vi "MAC-Tester.vi"() -> ()   [LabVIEW 2017]
uses:
  <vilib>/rvi/interface/nirviMethod/nirviMethod.xnode
  <vilib>/rvi/errors/niLvFpgaMergeErrorWithErrorCode.vi
  <vilib>/rvi/interface/nirviCloseFPGA/nirviCloseFPGA.xnode
  MAC.Events.ctl
  <vilib>/rvi/interface/nirviOpenFPGA/nirviOpenFPGA.xnode
  <vilib>/FPGAPlugInAG/Dynamic/niLvFpga_ReadFifo_Dynamic.vi
  <vilib>/FPGAPlugInAG/Dynamic/niLvFpga_WriteFifo_Dynamic.vi
  FPGA Bitfiles/Fpga-Mac-Top.lvbitx
  Globals.vi
  <vilib>/FPGAPlugInAG/Dynamic/niLvFpga_Close_Dynamic.vi
  <vilib>/FPGAPlugInAG/PXIe-6592R/niLvFpga_Open_PXIe-6592R.vi
  <vilib>/rvi/interface/common/dynamic/niFpgaDynamicAddResources.vi
panel:
  out "IPv4 Header":T1={"Version"=4, "Header Length"=20, "Total Length"=54, "More Fragments"=FALSE, "Don't Fragment"=FALSE, "Fragment Offset"=0, "TTL"=64, "Header Checksum"=58141, "Identification"=16593, "Protocol"=17} {"Header Checksum" format="%04x"}
  in  "IP Address":u8[](array[numeric])=[10, 0, 1, 101]
  in  "MAC":u8[](array[numeric])=[0, 1, 2, 3, 4, 5] format="%.0x"
  in  "Ethernet II Params":T2={"Destination MAC"=[0, 2, 201, 85, 8, 68], "Source MAC"=[0, 1, 2, 3, 4, 5], "EtherType"=2048} {"Destination MAC" format="%.0x"; "Source MAC" format="%.02x"; "EtherType" format="%.0x"}
  in  "IPv4 Params":T3={"Destination IP"=[10, 0, 1, 100], "Source IP"=[10, 0, 1, 101], "Protocol"=17}
  in  "UDP Params":T4={"Source Port"=35312, "Destination Port"=35312, "Payload"="ABCD"}
  out "Status":string
  out "error out":errorcluster
  in  "Exit":bool
  in  "Transmit Packet":bool
  in  "Read Packet":bool
  out "RX Data":u8[](array[numeric])=[0, 1, 2, 3, 4, 5, 0, 2, 201, 85, 8, 68, 8, 6, 0, 1, 8, 0, 6, 4, 0, 1, 0, 2, 201, 85, 8, 68, 10, 0, 1, 100, 0, 0, 0, 0, 0, 0, 10, 0, 1, 101, 0, 0, 0, 0, 0, 0, 0, 0, 0, 0, 0, 0, 0, 0, 0, 0, 0, 0, 28, 161, 25, 173] format="%.0x"
  in  "error in":errorcluster
  # "Send Parameters"
  # "Received Data"
  # "NIC Parameters"
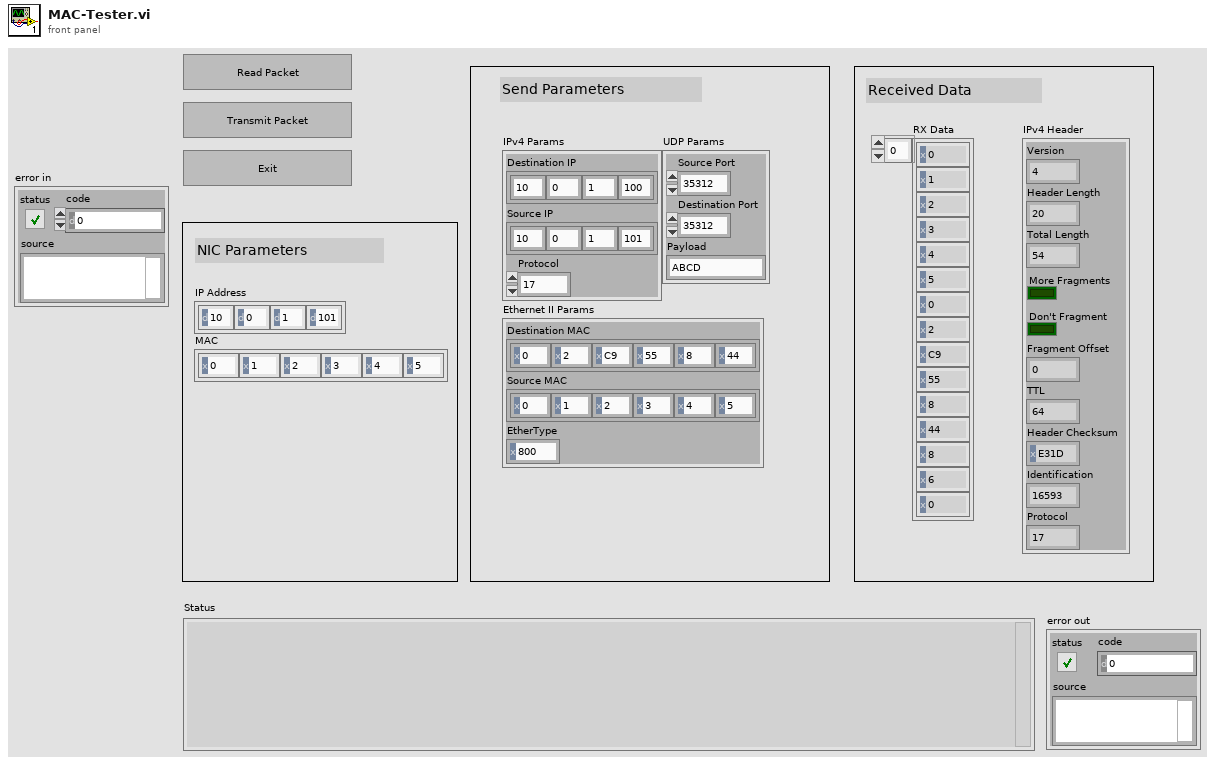
[diagram p1: front panel]
types:
  T1 = cluster{"Version":u8, "Header Length":u8, "Total Length":u16, "More Fragments":bool, "Don't Fragment":bool, "Fragment Offset":u16, "TTL":u8, "Header Checksum":u16, "Identification":u16, "Protocol":u8}
  T2 = cluster{"Destination MAC":u8[], "Source MAC":u8[], "EtherType":u16}
  T3 = cluster{"Destination IP":u8[], "Source IP":u8[], "Protocol":u8}
  T4 = cluster{"Source Port":u16, "Destination Port":u16, "Payload":string}
  T5 = typedef "MAC.Events.ctl" = enum16{"Open FPGA", "Close FPGA", "Poll RX", "Transmit Packet"}
  T6 = cluster{"Version":u8, "Header Length":u8, "Total Length":u16, "More Fragments":bool, "Don't Fragment":bool, "Fragment Offset":u16, "TTL":u8, "Header Checksum":u16, "Identification":u16, "Protocol":u8, "Source IP":u8[], "Destination IP":u8[]}
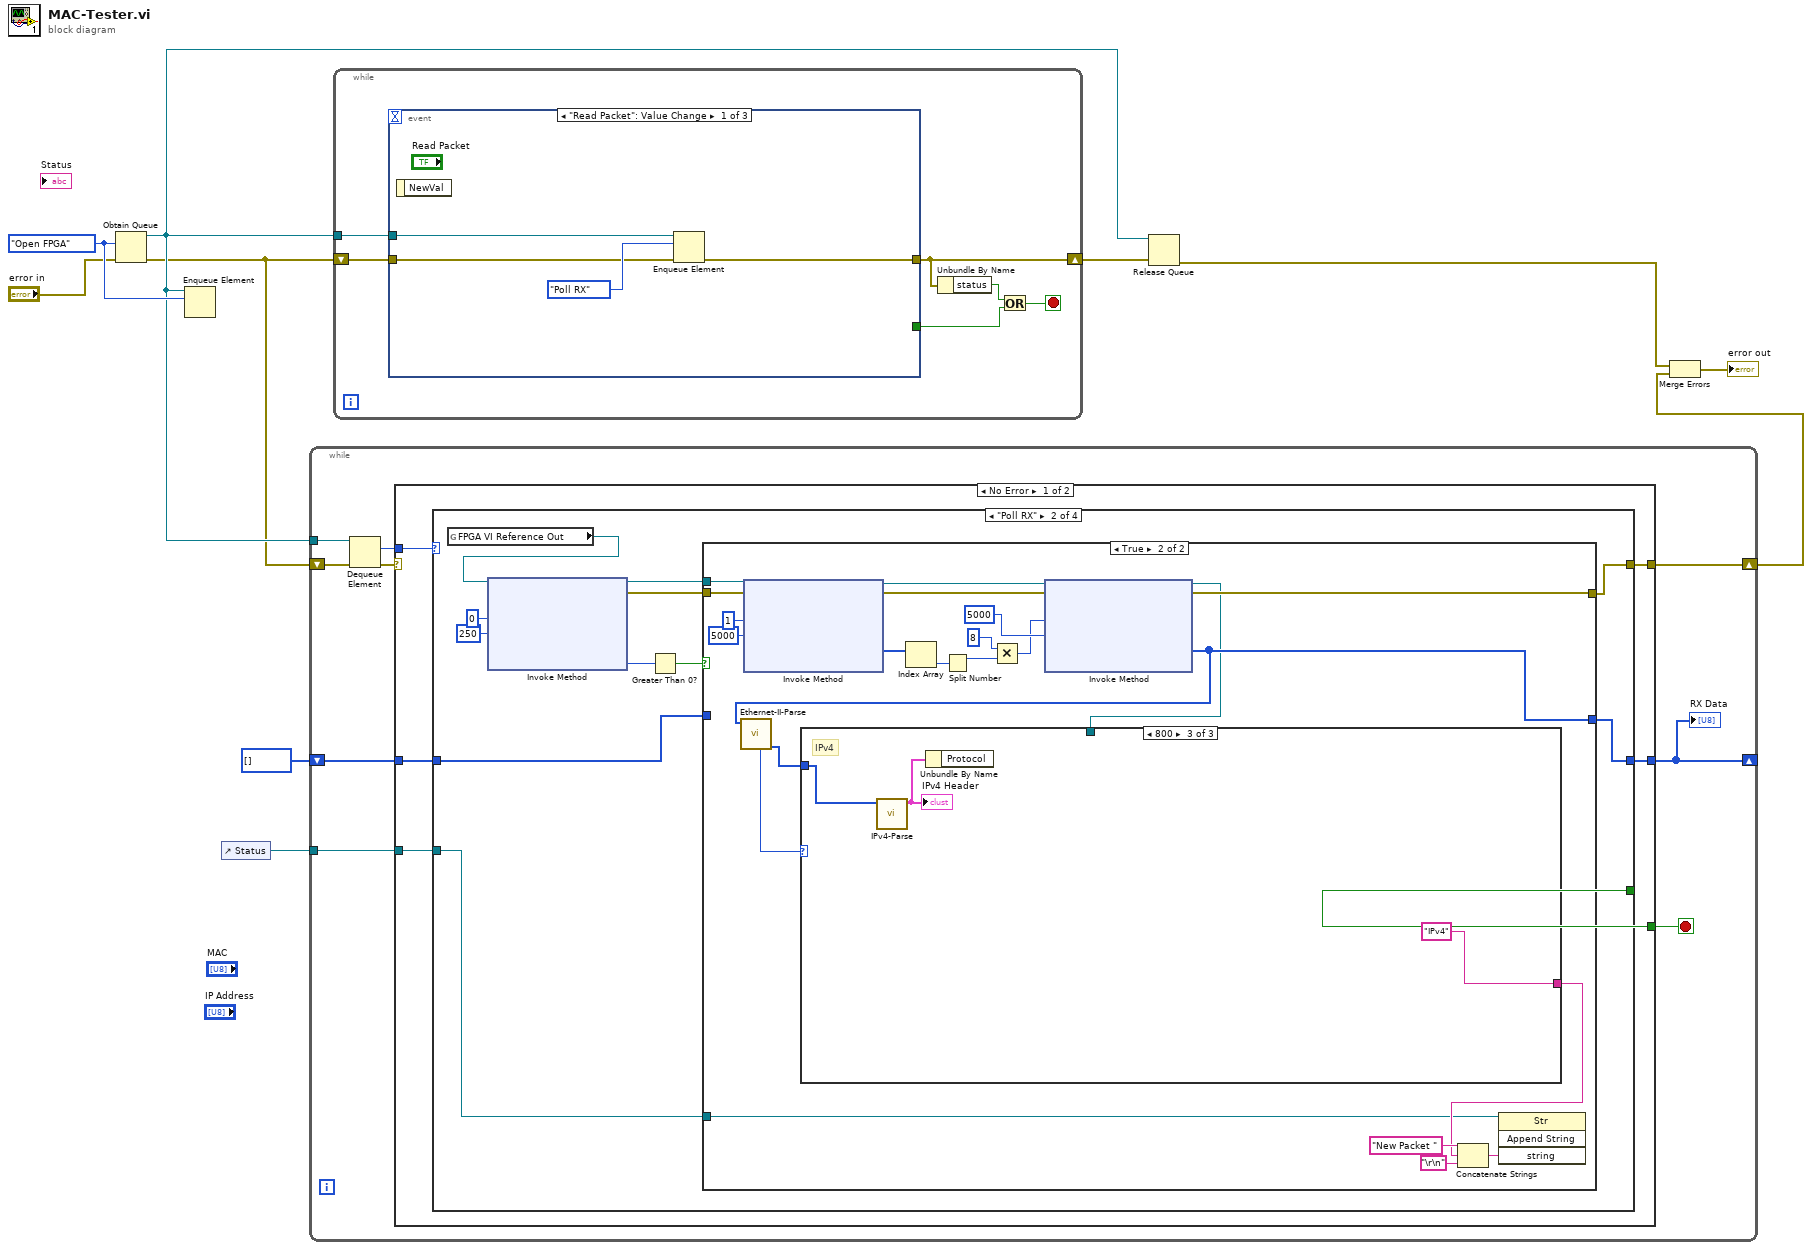
[diagram p0: block diagram]
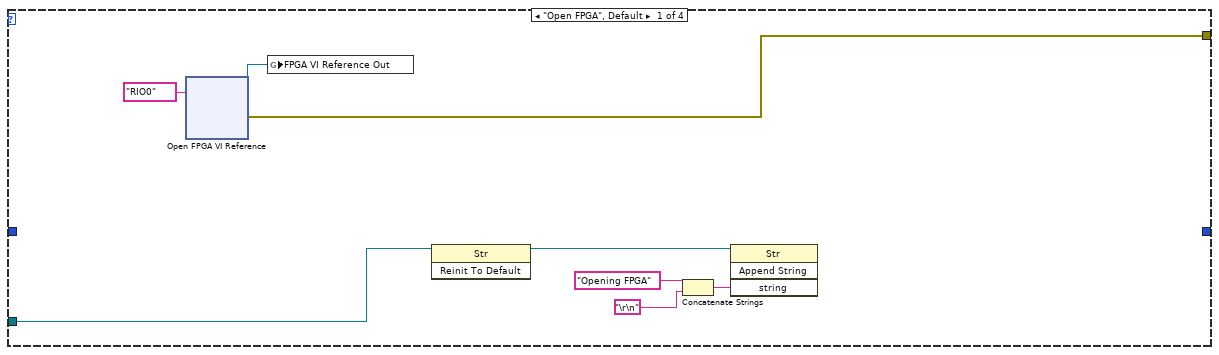
[diagram p2: hidden frame]
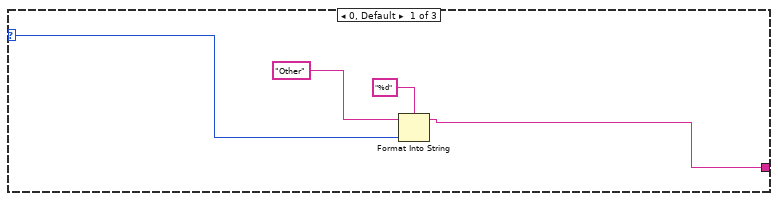
[diagram p4: hidden frame]
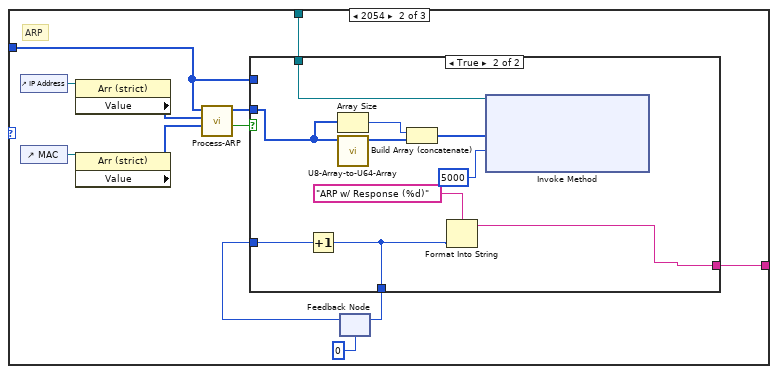
[diagram p5: hidden frame]
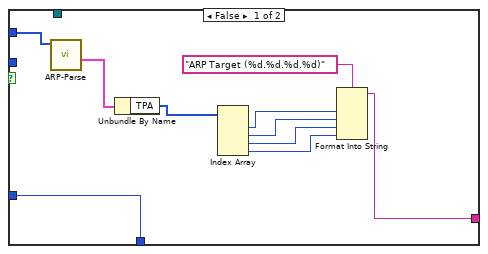
[diagram p6: hidden frame]
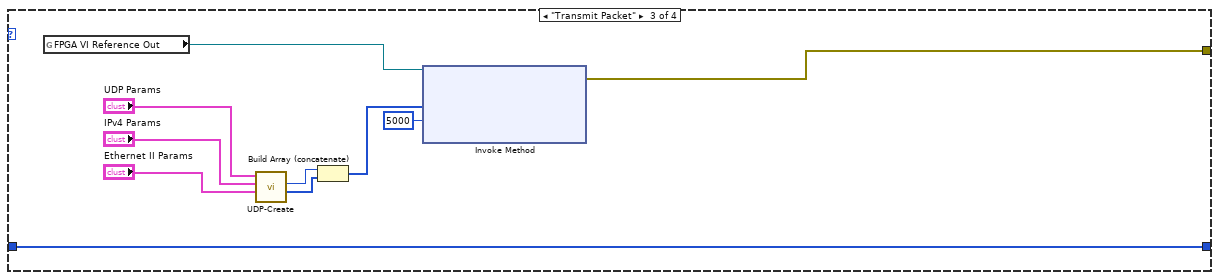
[diagram p7: hidden frame]
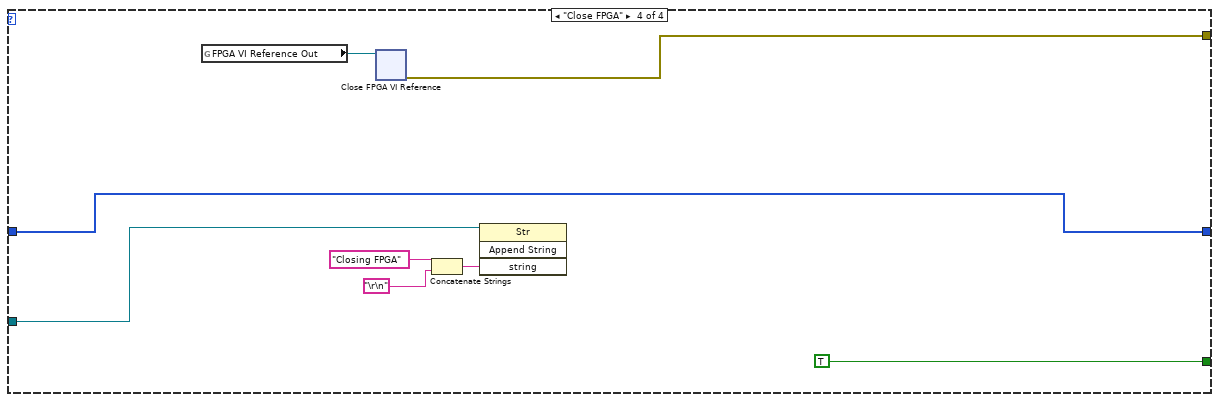
[diagram p8: hidden frame]
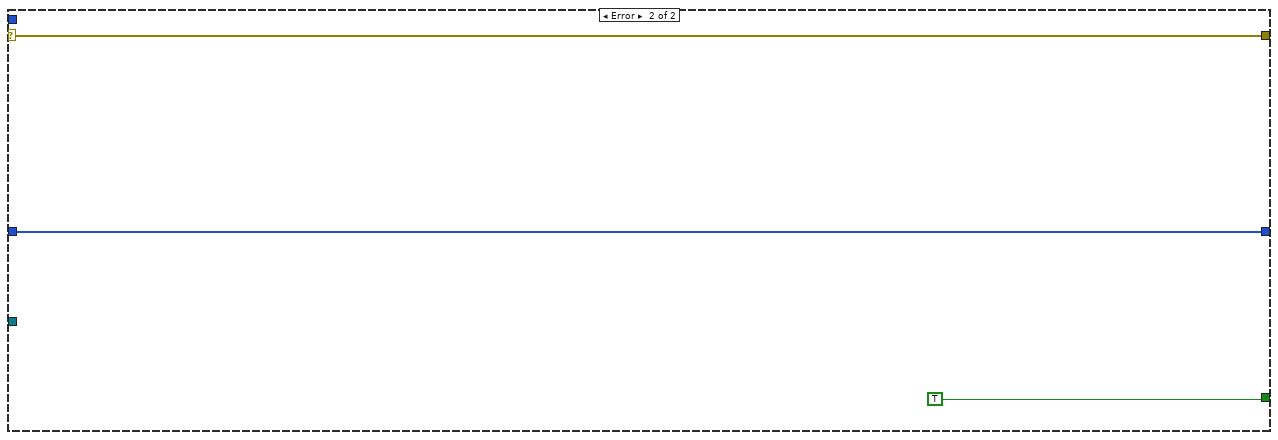
[diagram p9: hidden frame]
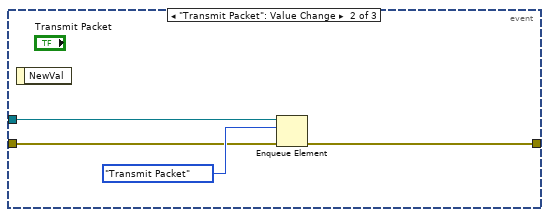
[diagram p10: hidden frame]
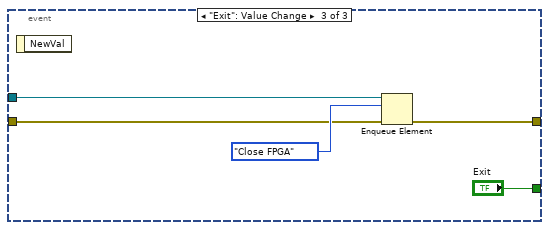
[diagram p11: hidden frame]
diagram:
  w10 = MAC.Events."Open FPGA"
  n1 = Obtain Queue(element data type=w10, error in (no error)="error in") -> (queue out=w8:refnum<queue>, error out=w6:errorcluster)  [unwired: 3 in, 1 out]
  n2 = Enqueue Element(queue=w8, element=w10) -> ()  [unwired: 2 in, 3 out]
  n3 = control-ref of="Status"() -> (w4:refnum<vi>)
  n4 = while {
    tunnel: w8 -> [w19]
    shift-right: [w13] -> w3
    shift-left: w6 -> [w15]
    shift-right: [w12] -> _
    shift-left: u8[] [] -> [w14]
    tunnel: w4 -> [w11]
    stop <- w16 stop-if-true
    n5 = Dequeue Element(queue=w19, error in (no error)=w15) -> (element=w17:T5, error out=w18:errorcluster)  [unwired: 1 in, 2 out]
    n6 = case shown="No Error" w18 {
      selector: w18 -> [_ w126]
      tunnel: w17 -> [w25 _]
      tunnel: [w24 TRUE] -> w16
      tunnel: [w23 w126] -> w13
      tunnel: w14 -> [w22 w127]
      tunnel: [w21 w127] -> w12
      tunnel: w11 -> [w20 _]
      frame No Error {
        n7 = case shown="\"Poll RX\"" w25 {
          tunnel: [_ _ _ TRUE] -> w24
          tunnel: [w33 w36 w109 w124] -> w23
          tunnel: w22 -> [_ w38 w117 w119]
          tunnel: [_ w37 w117 w119] -> w21
          tunnel: w20 -> [w29 w35 _ w120]
          frame "Open FPGA", Default {
            n8 = xnode "Open FPGA VI Reference"("resource name"=tag "RIO0") -> ("FPGA VI Reference Out"=w26:refnum<k20>, "error out"=w33:errorcluster)  [unwired: 1 in]
            n9 = global write "Globals.vi" "FPGA VI Reference Out"(w26) -> ()
            n10 = invoke class="Str" method="Reinit To Default"(reference=w29) -> (reference out=w28:refnum<vi>)  [unwired: 2 in, 2 out]
            n11 = Concatenate Strings("Opening FPGA" ("string"), "\r\n") -> (w32:string)
            n12 = invoke class="Str" method="Append String"(reference=w28, "string"=w32) -> ()  [unwired: 2 in, 4 out]
          }
          frame "Poll RX" {
            n13 = global read "Globals.vi" "FPGA VI Reference Out"() -> (w34:refnum<k20>)
            n14 = xnode "Invoke Method"("FPGA VI Reference In"=w34, "Number of Elements"=u32 0, "Timeout (ms)"=250) -> ("FPGA VI Reference Out"=w40:refnum<k20>, "error out"=w39:errorcluster, "Elements Remaining"=w42:u32)  [unwired: 1 in, 1 out]
            n15 = Greater Than 0?(x=w42) -> (x > 0?=w41:bool)
            n16 = case shown="True" w41 {
              tunnel: w40 -> [_ w66]
              tunnel: w39 -> [w45 w65]
              tunnel: w38 -> [w46 _]
              tunnel: [w46 w50] -> w37
              tunnel: [w45 w59] -> w36
              tunnel: w35 -> [_ w48]
              frame False {
              }
              frame True {
                n17 = xnode "Invoke Method"("FPGA VI Reference In"=w66, "error in"=w65, "Number of Elements"=u32 1, "Timeout (ms)"=5000) -> ("FPGA VI Reference Out"=w62:refnum<k20>, "error out"=w63:errorcluster, "Data"=w64:u32[])  [unwired: 1 out]
                n18 = Index Array(array=w64) -> (element=w61:u32)  [unwired: 1 in]
                n19 = Split Number(x=w61) -> (hi(x)=w55:u16)  [unwired: 1 out]
                n20 = Multiply(x=u16 8 ("y"), y=w55) -> (x*y=w58:u16)
                n21 = xnode "Invoke Method"("FPGA VI Reference In"=w62, "error in"=w63, "Number of Elements"=w58, "Timeout (ms)"=5000) -> ("FPGA VI Reference Out"=w49:refnum<k20>, "error out"=w59:errorcluster, "Data"=w50:u8[])  [unwired: 1 out]
                n22 = call "Ethernet-II-Parse.vi"("Input Frame"=w50) -> ("Payload"=w47:u8[], "EtherType"=w53:u16)  [unwired: 6 in, 3 out]
                n23 = case shown="800" w53 {
                  selector: w53 -> [w72 _ _]
                  tunnel: [w69 w80 "IPv4" ("string")] -> w51
                  tunnel: w47 -> [_ w73 w106]
                  tunnel: w49 -> [_ w77 _]
                  frame 0, Default {
                    n24 = Format Into String(format string="%d", initial string="Other" ("string"), w72) -> (resulting string=w69:string)  [unwired: 1 in, 1 out]
                  }
                  frame 2054 {
                    # "ARP"
                    n25 = control-ref of="IP Address"() -> (w82:refnum<vi>)
                    n26 = control-ref of="MAC"() -> (w84:refnum<vi>)
                    n27 = property class="Arr (strict)"(reference=w82) -> ("Value"=w81:u8[])  [unwired: 1 in, 2 out]
                    n28 = property class="Arr (strict)"(reference=w84) -> ("Value"=w83:u8[])  [unwired: 1 in, 2 out]
                    n29 = call "Process-ARP.vi"(9:w83, "Source Machine\nSettings"=w81, "Frame (in)"=w73) -> ("Response\nNeeded?"=w79:bool, "ARP Response"=w78:u8[])  [unwired: 7 in]
                    n30 = feedback #1(0) -> (w74:i32)
                    n31 = case shown="True" w79 {
                      tunnel: [w91 w95] -> w80
                      tunnel: w78 -> [_ w102]
                      tunnel: w77 -> [_ w103]
                      tunnel: [w94 w97] -> w75
                      tunnel: w74 -> [w94 w98]
                      tunnel: w73 -> [w93 _]
                      frame False {
                        n32 = call "ARP-Parse.vi"("Frame (in)"=w93) -> ("Target"=w90:cluster{"THA":u8[], "TPA":u8[]})  [unwired: 8 in, 2 out]
                        n33 = Unbundle By Name(w90) -> ("TPA"=w89:u8[])
                        n34 = Index Array(array=w89) -> (element #1=w88:u8, element #2=w85:u8, element #3=w86:u8, element #4=w87:u8)  [unwired: 4 in]
                        n35 = Format Into String(format string="ARP Target (%d.%d.%d.%d)", w88, w85, w86, w87) -> (resulting string=w91:string)  [unwired: 2 in, 1 out]
                      }
                      frame True {
                        n36 = Increment(x=w98) -> (x+1=w97:i32)
                        n37 = Array Size(array=w102) -> (size(s)=w100:i32)
                        n38 = call "U8-Array-to-U64-Array.vi"("Frame U8[] in"=w102) -> ("Frame U64[] out"=w101:u64[])  [unwired: 10 in]
                        n39 = Build Array (concatenate)(w100, w101) -> (w99:u64[])
                        n40 = Format Into String(format string="ARP w/ Response (%d)", w97) -> (resulting string=w95:string)  [unwired: 2 in, 1 out]
                        n41 = xnode "Invoke Method"("FPGA VI Reference In"=w103, "Data"=w99, "Timeout (ms)"=5000) -> ()  [unwired: 1 in, 3 out]
                      }
                    }
                    n42 = feedback-in #1(w75) -> ()
                  }
                  frame 2048 {
                    # "IPv4"
                    n43 = call "IPv4-Parse.vi"("IPv4 Packet (in)"=w106) -> ("Header"=w105:T6)  [unwired: 8 in, 2 out]
                    "IPv4 Header" <- w105
                    n44 = Unbundle By Name(w105) -> ()  [unwired: 1 out]
                  }
                }
                n45 = Concatenate Strings("New Packet " ("string"), w51, "\r\n") -> (w57:string)
                n46 = invoke class="Str" method="Append String"(reference=w48, "string"=w57) -> ()  [unwired: 2 in, 4 out]
              }
            }
          }
          frame "Transmit Packet" {
            n47 = global read "Globals.vi" "FPGA VI Reference Out"() -> (w108:refnum<k20>)
            n48 = call "UDP-Create.vi"("Ethernet II Params"="Ethernet II Params", "IPv4 Params"="IPv4 Params", "UDP Params"="UDP Params") -> ("Ethernet Frame\nU64"=w112:u64[], "Ethernet Frame\nsize"=w113:i32)  [unwired: 6 in, 1 out]
            n49 = Build Array (concatenate)(w113, w112) -> (w111:u64[])
            n50 = xnode "Invoke Method"("FPGA VI Reference In"=w108, "Data"=w111, "Timeout (ms)"=5000) -> ("error out"=w109:errorcluster)  [unwired: 1 in, 2 out]
          }
          frame "Close FPGA" {
            n51 = global read "Globals.vi" "FPGA VI Reference Out"() -> (w118:refnum<k20>)
            n52 = xnode "Close FPGA VI Reference"("FPGA VI Reference In"=w118) -> ("error out"=w124:errorcluster)  [unwired: 1 in]
            n53 = Concatenate Strings("Closing FPGA" ("string"), "\r\n") -> (w123:string)
            n54 = invoke class="Str" method="Append String"(reference=w120, "string"=w123) -> ()  [unwired: 2 in, 4 out]
          }
        }
      }
      frame Error {
      }
    }
    "RX Data" <- w12
  }
  n55 = while {
    tunnel: w8 -> [w134]
    shift-right: [w129] -> w9
    shift-left: w6 -> [w130]
    stop <- w132 stop-if-true
    n56 = event shown="[0] \"Read Packet\": Value Change" {
      selector: _ -> [_ _ _]
      dyn-events: _ -> [_ _ _]
      timeout: _ -> [_ _ _]
      tunnel: w134 -> [w138 w141 w146]
      tunnel: [w136 w139 w145] -> w129
      tunnel: [_ _ "Exit"] -> w131
      tunnel: w130 -> [w135 w140 w143]
      event "Read Packet": Value Change {
        n57 = event-data() -> ()  [unwired: 1 in, 1 out]
        n58 = Enqueue Element(queue=w138, element=MAC.Events."Poll RX", error in (no error)=w135) -> (error out=w136:errorcluster)  [unwired: 1 in, 2 out]
      }
      event "Transmit Packet": Value Change {
        n59 = event-data() -> ()  [unwired: 1 in, 1 out]
        n60 = Enqueue Element(queue=w141, element=MAC.Events."Transmit Packet", error in (no error)=w140) -> (error out=w139:errorcluster)  [unwired: 1 in, 2 out]
      }
      event "Exit": Value Change {
        n61 = event-data() -> ()  [unwired: 1 in, 1 out]
        n62 = Enqueue Element(queue=w146, element=MAC.Events."Close FPGA", error in (no error)=w143) -> (error out=w145:errorcluster)  [unwired: 1 in, 2 out]
      }
    }
    n63 = Unbundle By Name(w129) -> ("status"=w133:bool)
    n64 = Or(x=w133, y=w131) -> (x .or. y?=w132:bool)
  }
  n65 = Release Queue(queue=w8, error in (no error)=w9) -> (error out=w1:errorcluster)  [unwired: 1 in, 2 out]
  n66 = Merge Errors(w1, w3) -> (→"error out":errorcluster)
